vi "PCM Generation with Master Clock.vi"() -> ()   [LabVIEW 2021]
uses:
  <vilib>/PDM Acquisition Toolkit/host/API/Controls/Generation State.ctl
  <vilib>/PDM Acquisition Toolkit/shared/controls/clock mode.ctl
  <vilib>/PDM Acquisition Toolkit/shared/controls/PCM Frame Sync Control.ctl
  <vilib>/PDM Acquisition Toolkit/shared/controls/Digital Edge.ctl
  <vilib>/PDM Acquisition Toolkit/shared/controls/PCM Data Format Configuration.ctl
  <vilib>/PDM Acquisition Toolkit/shared/controls/PCM Bit Endianness.ctl
  <vilib>/PDM Acquisition Toolkit/shared/controls/PCM Data Justification.ctl
  <vilib>/PDM Acquisition Toolkit/host/Classes/Session/Controls/Logic Levels.ctl
  <vilib>/PDM Acquisition Toolkit/host/API/Controls/PDM Digital Start Trigger Cluster.ctl
  <vilib>/PDM Acquisition Toolkit/shared/controls/PXI trigger lines.ctl
  <vilib>/PDM Acquisition Toolkit/shared/controls/trigger polarity.ctl
  <vilib>/PDM Acquisition Toolkit/host/API/Public/Function Generator/Configure Custom Signal (N Ch) - PCM Output Task.vi
  <vilib>/PDM Acquisition Toolkit/host/API/Public/Configure/Triggering/Configure PCM Output Trigger (Digital Edge).vi
  <vilib>/PDM Acquisition Toolkit/shared/PDM Shared.lvlib
  <vilib>/PDM Acquisition Toolkit/host/API/PDM Acquisition Toolkit.lvlib
  <vilib>/PDM Acquisition Toolkit/host/Classes/Session/DecoderSession.lvclass
panel:
  in  "Trigger Generation":bool
  in  "Invert Frame Clock":bool
  in  "MSB First":bool
  in  "Bit Clock Edge Sync":enum16{"Rising", "Falling"}(ring)
  in  "Number of Channels":u16=2
  in  "Logic Level":enum16{"3.3", "1.8", "1.2"}(ring)
  in  "Channel Length":u16=32
  in  "Bit Depth":u8=24
  in  "Frame Clock Rate":sgl=48000.0 format="%#_6pHz"
  in  "Justification":enum16{"Left", "Right"}(ring)
  in  "Master Clock Rate":sgl=12288000.0 format="%#_6pHz"
  in  "Master Clk line":string="7821\\PCMo 0"
  out "Error Out":errorcluster
  in  "Tab Control":enum32{"Custom Signal"}(tab)
  in  "phase":dbl caption="phase 2"
  in  "gain":dbl=0.5
  in  "frequency":dbl=1000.0 caption="frequency - custom"
  in  "signal type":T1(ring)
  out "Bit Clock Rate":sgl=3072000.0 format="%#_6pHz"
  in  "Stop":bool
  out "state":T2=enum."Active"
  in  "channel list":string="7821\\PCMo 8"
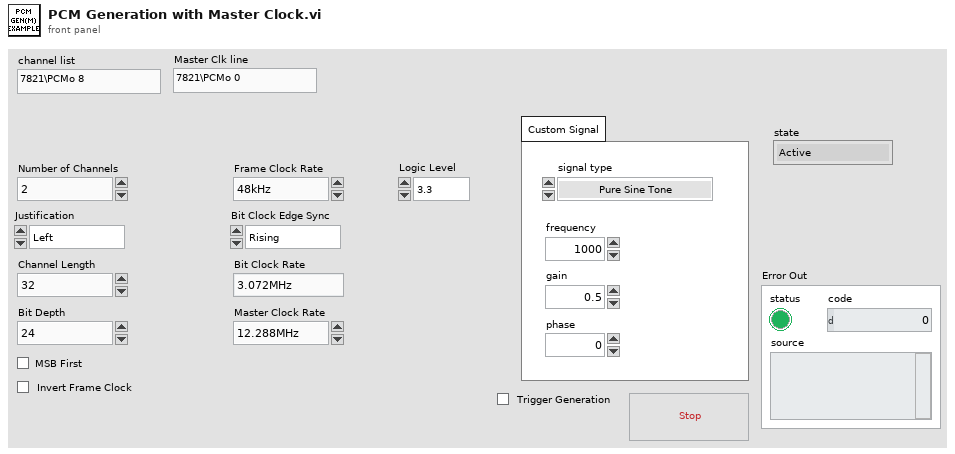
[diagram p1: front panel]
types:
  T1 = enum16{"Pure Sine Tone", "Triangular Wave", "Dual Tone 10kHz - 11kHz", "Multisine 22 Tones", "Multisine 200 Tones", "SMPTE 60-7000 Hz"}
  T2 = typedef "PDM Acquisition Toolkit.lvlib/Generation State.ctl" = enum16{"Idle", "Waiting on Trigger", "Active"}
  T3 = typedef "PDM Shared.lvlib/PCM Data Format Configuration.ctl" = cluster{"Frame Sync Edge for Channel 0":T4, "Channel Count Per Frame":u8, "Channel Length":u16, "Bit Depth":u8, "Channel 0 Offset":u16, "Endianness":T5, "Data Justification":T6}
  T4 = typedef "PDM Shared.lvlib/Digital Edge.ctl" = enum8{"Rising", "Falling"}
  T5 = typedef "PDM Shared.lvlib/PCM Bit Endianness.ctl" = enum16{"MSB First", "LSB First"}
  T6 = typedef "PDM Shared.lvlib/PCM Data Justification.ctl" = enum16{"Left Justified", "Right Justified"}
  T7 = typedef "PDM Shared.lvlib/PCM Frame Sync Control.ctl" = cluster{"Frame Length":u16, "Frame Sync Pulse Width":u16, "Bit Clock Edge  Sync":T4}
  T8 = typedef "PDM Shared.lvlib/clock mode.ctl" = enum16{"divided clock", "DDS"}
  T9 = typedef "PDM Acquisition Class Library.lvlib/DecoderSession.lvclass/Logic Levels.ctl" = enum16{"3.3 V", "1.8 V", "1.2 V"}
  T10 = typedef "PDM Acquisition Class Library.lvlib/PCM Output Task.lvclass/PCM Output Task DVR.ctl" = refnum<data-value>
  T11 = typedef "PDM Acquisition Class Library.lvlib/I2S Output Task.lvclass/SignalProperties.ctl" = cluster{"cyclic signal":dbl[], "channel parameters":T12[]}
  T12 = typedef "PDM Acquisition Class Library.lvlib/I2S Output Channel.lvclass/GenerationChannelProperties.ctl" = cluster{"cyclic period":dbl, "cyclic phase offset":dbl, "gain":dbl}
  T13 = typedef "PDM Acquisition Toolkit.lvlib/PDM Digital Start Trigger Cluster.ctl" = cluster{"source":T14, "polarity":T15}
  T14 = typedef "PDM Shared.lvlib/PXI trigger lines.ctl" = enum16{"PXI_Trig0", "PXI_Trig1", "PXI_Trig2", "PXI_Trig3", "PXI_Trig4", "PXI_Trig5", "PXI_Trig6", "PXI_Trig7"}
  T15 = typedef "PDM Shared.lvlib/trigger polarity.ctl" = enum16{"Rising Edge", "Falling Edge"}
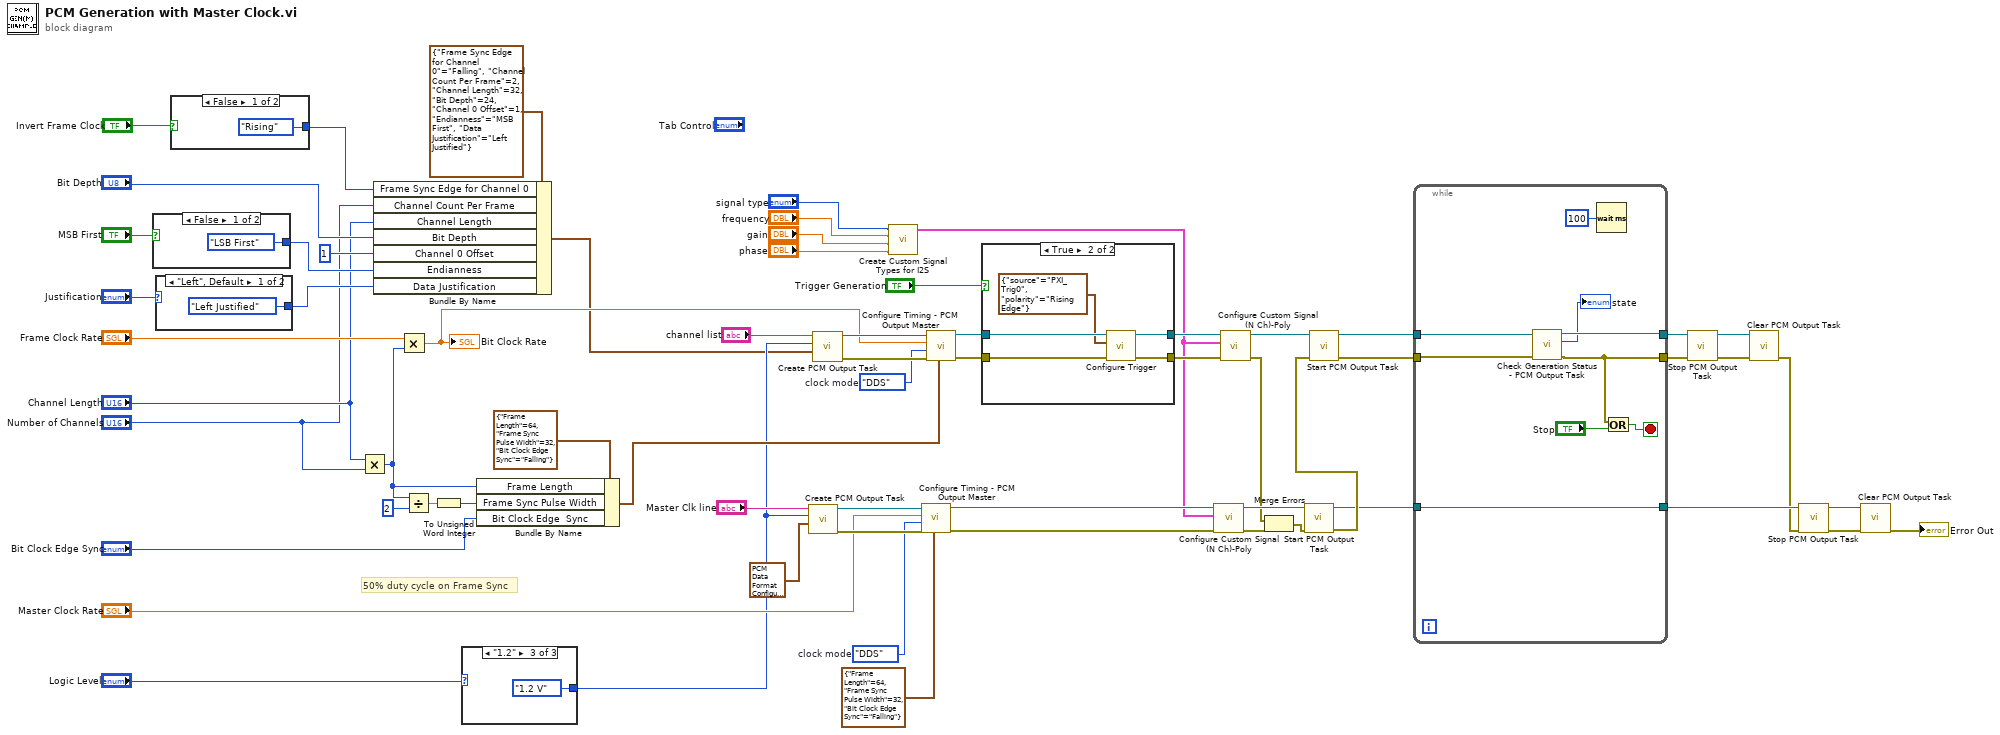
[diagram p0: block diagram]
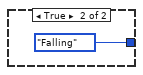
[diagram p3: hidden frame]
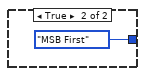
[diagram p4: hidden frame]
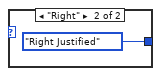
[diagram p5: hidden frame]
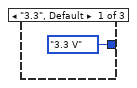
[diagram p6: hidden frame]
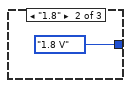
[diagram p7: hidden frame]
diagram:
  w50 = clock_mode."DDS"  # clock mode
  w55 = clock_mode."DDS"  # clock mode
  # "50% duty cycle on Frame Sync"
  n1 = case shown="False" "MSB First" {
    tunnel: [PCM_Bit_Endianness."LSB First" ("Endianness") PCM_Bit_Endianness."MSB First" ("Endianness")] -> w24
    frame False {
    }
    frame True {
    }
  }
  n2 = case shown="\"Left\", Default" "Justification" {
    tunnel: [PCM_Data_Justification."Left Justified" ("Data Justification") PCM_Data_Justification."Right Justified" ("Data Justification")] -> w26
    frame "Left", Default {
    }
    frame "Right" {
    }
  }
  n3 = case shown="False" "Invert Frame Clock" {
    tunnel: [Digital_Edge."Rising" ("Frame Sync Edge for Channel 0") Digital_Edge."Falling" ("Frame Sync Edge for Channel 0")] -> w19
    frame False {
    }
    frame True {
    }
  }
  n4 = Multiply(x="Channel Length", y="Number of Channels") -> (x*y=w30:u16)
  n5 = Bundle By Name(cluster=T3 {"Frame Sync Edge for Channel 0"=enum."Falling", "Channel Count Per Frame"=2, "Channel Length"=32, "Bit Depth"=24, "Channel 0 Offset"=1, "Endianness"=enum."MSB First", "Data Justification"=enum."Left Justified"} ("PCM Data Configuration"), "Frame Sync Edge for Channel 0"=w19, "Channel Count Per Frame"="Number of Channels", "Channel Length"="Channel Length", "Bit Depth"="Bit Depth", "Channel 0 Offset"=u16 1, "Endianness"=w24, "Data Justification"=w26) -> (w27:T3)
  n6 = Multiply(x="Frame Clock Rate", y=w30) -> (x*y=w29:sgl)
  "Bit Clock Rate" <- w29
  n7 = Divide(x=w30, y=u16 2) -> (x/y=w35:dbl)
  n8 = To Unsigned Word Integer(number=w35) -> (unsigned 16bit integer=w34:u16)
  n9 = case shown="\"1.2\"" "Logic Level" {
    tunnel: [Logic_Levels."3.3 V" ("logic level") Logic_Levels."1.8 V" ("logic level") Logic_Levels."1.2 V" ("logic level")] -> w33
    frame "3.3", Default {
    }
    frame "1.8" {
    }
    frame "1.2" {
    }
  }
  n10 = Bundle By Name(cluster=T7 {"Frame Length"=64, "Frame Sync Pulse Width"=32, "Bit Clock Edge  Sync"=enum."Falling"} ("Frame Sync Clock Control"), "Frame Length"=w30, "Frame Sync Pulse Width"=w34, "Bit Clock Edge  Sync"="Bit Clock Edge Sync") -> (w38:T7)
  n11 = call <vilib>:"Create PCM Output Task.vi"("PCM data configuration"=T3 {"Frame Sync Edge for Channel 0"=enum."Falling", "Channel Count Per Frame"=2, "Channel Length"=32, "Bit Depth"=24, "Channel 0 Offset"=1, "Endianness"=enum."MSB First", "Data Justification"=enum."Left Justified"} ("PCM Data Configuration 2"), "logic level"=w33, "channel list"="Master Clk line") -> ("error out"=w52:errorcluster, "PCM output task out"=w53:T10)  [unwired: 7 in]
  n12 = call <vilib>:"Create PCM Output Task.vi"("PCM data configuration"=w27, "logic level"=w33, "channel list"="channel list") -> ("error out"=w56:errorcluster, "PCM output task out"=w57:T10)  [unwired: 7 in]
  n13 = call "Create Custom Signal Types for I2S.vi"("phase"="phase", "gain"="gain", "frequency"="frequency", "signal type"="signal type") -> ("Signal Properties"=w5:T11)  [unwired: 7 in]
  n14 = call <vilib>:"Configure Timing - PCM Output Master.vi"("Frame Sync Clock Control"=T7 {"Frame Length"=64, "Frame Sync Pulse Width"=32, "Bit Clock Edge  Sync"=enum."Falling"} ("Frame Sync Clock Control 2"), "error in"=w52, "clock mode"=w50, "Bit Clock rate"="Master Clock Rate", "PCM output task in"=w53) -> ("error out"=w13:errorcluster, "PCM output task out"=w12:T10)  [unwired: 4 in, 1 out]
  n15 = call <vilib>:"Configure Timing - PCM Output Master.vi"("Frame Sync Clock Control"=w38, "error in"=w56, "clock mode"=w55, "Bit Clock rate"=w29, "PCM output task in"=w57) -> ("error out"=w16:errorcluster, "PCM output task out"=w17:T10)  [unwired: 4 in, 1 out]
  n16 = case shown="True" "Trigger Generation" {
    tunnel: w17 -> [w75 w80]
    tunnel: w16 -> [w74 w79]
    tunnel: [w75 w78] -> w9
    tunnel: [w74 w77] -> w10
    frame False {
    }
    frame True {
      n17 = call-poly <vilib>:"Configure Trigger.vi"("error in"=w79, "trigger configuration"=T13 {"source"=enum."PXI_Trig0", "polarity"=enum."Rising Edge"}, "PCM output task in"=w80) -> ("error out"=w77:errorcluster, "PCM output task out"=w78:T10)  [unwired: 7 in]
    }
  }
  n18 = call-poly <vilib>:"Configure Custom Signal (N Ch)-Poly.vi"("error in"=w13, "signal parameters"=w5, "PCM output task in"=w12) -> ("error out"=w6:errorcluster, "PCM output task out"=w11:T10)  [unwired: 7 in]
  n19 = call-poly <vilib>:"Configure Custom Signal (N Ch)-Poly.vi"("error in"=w10, "signal parameters"=w5, "PCM output task in"=w9) -> ("error out"=w7:errorcluster, "PCM output task out"=w8:T10)  [unwired: 7 in]
  n20 = Merge Errors(w7, w6) -> (w46:errorcluster)
  n21 = call <vilib>:"Start PCM Output Task.vi"("error in"=w46, "PCM output task in"=w11) -> ("error out"=w47:errorcluster, "PCM output task out"=w43:T10)  [unwired: 8 in]
  n22 = call <vilib>:"Start PCM Output Task.vi"("error in"=w47, "PCM output task in"=w8) -> ("error out"=w58:errorcluster, "PCM output task out"=w61:T10)  [unwired: 8 in]
  n23 = while {
    tunnel: w61 -> [w85]
    tunnel: [w84] -> w60
    tunnel: [w83] -> w59
    tunnel: w58 -> [w86]
    tunnel: w43 -> [w81]
    tunnel: [w81] -> w42
    stop <- w88 stop-if-true
    n24 = call <vilib>:"Check Generation Status - PCM Output Task.vi"("error in"=w86, "PCM output task in"=w85) -> ("error out"=w83:errorcluster, "state"=→"state":T2, "PCM output task out"=w84:T10)  [unwired: 6 in, 1 out]
    n25 = Wait (ms)(milliseconds to wait=u32 100) -> ()  [unwired: 1 out]
    n26 = Or(x=w83, y="Stop") -> (x .or. y?=w88:bool)
  }
  n27 = call <vilib>:"Stop PCM Output Task.vi"("error in"=w59, "PCM output task In"=w60) -> ("error out"=w64:errorcluster, "PCM output task out"=w63:T10)  [unwired: 8 in]
  n28 = call <vilib>:"Clear PCM Output Task.vi"("error in"=w64, "PCM output task in"=w63) -> ("error out"=w41:errorcluster)  [unwired: 9 in]
  n29 = call <vilib>:"Stop PCM Output Task.vi"("error in"=w41, "PCM output task In"=w42) -> ("error out"=w45:errorcluster, "PCM output task out"=w44:T10)  [unwired: 8 in]
  n30 = call <vilib>:"Clear PCM Output Task.vi"("error in"=w45, "PCM output task in"=w44) -> ("error out"=→"Error Out":errorcluster)  [unwired: 9 in]
